vi "TDS_Trigger_GetLevel.vi"(6 "TriggerSource":string, 8 "error in":errorcluster, 11 "VI Server Cluster":T1) -> (0 "error out":errorcluster, 1 "TriggerLevel (V)":dbl, 3 "VI Server Cluster DUP":T1)   [LabVIEW 2020]
uses:
  <vilib>/Utility/config.llb/NI_LVConfig.lvlib
  <vilib>/Utility/config.llb/Read Key (Double).vi
  NA-E5071B/E5071B.llb/Recover Variant.vi
  NA-E5071B/E5071B.llb/Recover Text Ring DBL.vi
  NA-E5071B/E5071B.llb/Labels&Control References.ctl
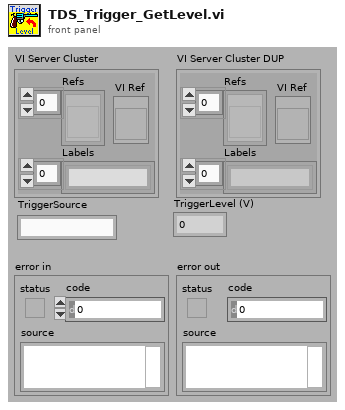
[diagram p1: front panel]
types:
  T1 = typedef "Labels&Control References.ctl" = cluster{"Refs":refnum<vi>[], "Labels":string[], "VI Ref":refnum<vi>}
  T2 = typedef "NI_LVConfig.lvlib/Config Data RefNum.ctl" = refnum<k1>
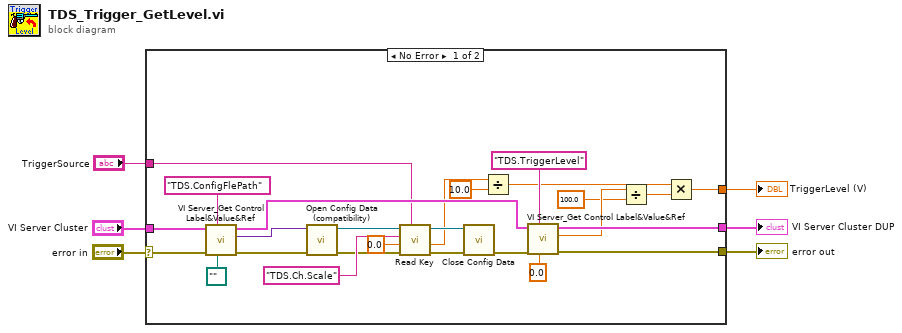
[diagram p0: block diagram]
diagram:
  n1 = case shown="No Error" "error in" {
    selector: "error in" -> [w14 w33]
    tunnel: "VI Server Cluster" -> [w32 _]
    tunnel: [w31 _] -> w5
    tunnel: [w29 w33] -> w4
    tunnel: [w15 _] -> w3
    tunnel: "TriggerSource" -> [w11 _]
    frame No Error {
      n2 = call-poly "VI Server_Get Control Label&Value&Ref.vi"("Default Value (Variant)"=path "" ("TDS.ConfigFlePath"), "Label"="TDS.ConfigFlePath", "error in"=w14, "Data Cluster"=w32) -> ("error out"=w23:errorcluster, "Value (Variant)"=w7:variant, "Data Cluster dup"=w30:T1)  [unwired: 3 in, 2 out]
      n3 = call <vilib>:"Open Config Data (compatibility).vi"("error in (no error)"=w23, "configuration file path"=w7) -> ("error out"=w13:errorcluster, "refnum"=w12:T2)  [unwired: 7 in, 1 out]
      n4 = call-poly <vilib>:"Read Key.vi"("section"=w11, "error in (no error)"=w13, "default value"=0.0, "key"="TDS.Ch.Scale", "refnum"=w12) -> ("error out"=w26:errorcluster, "value"=w16:dbl, "refnum out"=w27:T2)  [unwired: 3 in, 1 out]
      n5 = call <vilib>:"Close Config Data.vi"("error in (no error)"=w26, "refnum"=w27) -> ("error out"=w28:errorcluster)  [unwired: 8 in, 1 out]
      n6 = Divide(x=w16, y=10.0) -> (x/y=w10:dbl)
      n7 = call-poly "VI Server_Get Control Label&Value&Ref.vi"("Default Value"=0.0 ("TDS.TriggerLevel"), "Label"="TDS.TriggerLevel", "error in"=w28, "Data Cluster"=w30) -> ("error out"=w29:errorcluster, "Value"=w19:dbl, "Data Cluster dup"=w31:T1)  [unwired: 3 in, 2 out]
      n8 = Divide(x=w19, y=100.0) -> (x/y=w17:dbl)
      n9 = Multiply(x=w10, y=w17) -> (x*y=w15:dbl)
    }
    frame Error {
    }
  }
  "VI Server Cluster DUP" <- w5
  "error out" <- w4
  "TriggerLevel (V)" <- w3
